vi "UnitsToCounts.vi"(7 "Units (Encoder Counts)":T1=enum."Encoder Counts", 9 "Gear Ratio":dbl, 10 "Counts/Rev":dbl, 11 "Value":dbl) -> (5 "Encoder Counts":dbl)   [LabVIEW 2010]
uses:
  Typedefs/Units_Enum.ctl
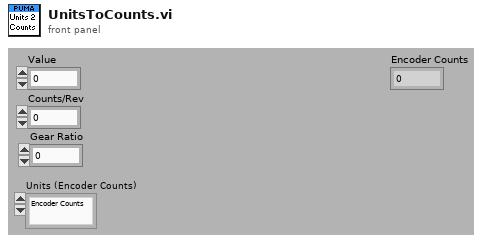
[diagram p1: front panel]
types:
  T1 = typedef "Units_Enum.ctl" = enum16{"Radians", "Encoder Counts", "Revolutions", "Degrees"}
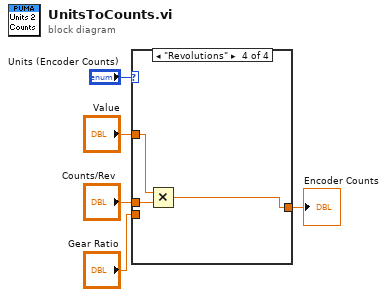
[diagram p0: block diagram]
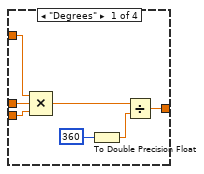
[diagram p2: hidden frame]
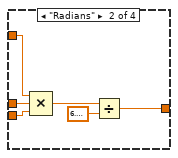
[diagram p3: hidden frame]
diagram:
  n1 = case shown="\"Revolutions\"" "Units (Encoder Counts)" {
    tunnel: [w11 w17 w19 w22] -> w3
    tunnel: "Value" -> [w6 w13 w19 w21]
    tunnel: "Counts/Rev" -> [w8 w15 _ w20]
    tunnel: "Gear Ratio" -> [w7 w14 _ _]
    frame "Degrees" {
      n2 = Compound Arithmetic op=MULTIPLY(w6, w8, w7) -> (w12:dbl)
      n3 = To Double Precision Float(number=360) -> (double precision float=w9:dbl)
      n4 = Divide(x=w12, y=w9) -> (x/y=w11:dbl)
    }
    frame "Radians" {
      n5 = Compound Arithmetic op=MULTIPLY(w13, w15, w14) -> (w18:dbl)
      n6 = Divide(x=w18, y=6.283185307179586) -> (x/y=w17:dbl)
    }
    frame "Encoder Counts", Default {
    }
    frame "Revolutions" {
      n7 = Multiply(x=w21, y=w20) -> (x*y=w22:dbl)
    }
  }
  "Encoder Counts" <- w3
